vi "Save Enabled Settings.vi"(8 "Error in":errorcluster caption="Error in (no error)", 10 "Enabled Sections":T1={"Projects"=TRUE, "Interfaces"=TRUE, "Classes"=TRUE, "Libraries"=TRUE, "VIs"=TRUE, "Controls"=TRUE, "LLBs"=TRUE}, 11 "Settings Path":path) -> (0 "Error out":errorcluster)   [LabVIEW 2023, in "VIDoc Printer.lvlib" / "Printer Settings.lvclass"]
uses:
  Printer Settings.lvclass
  Enabled Sections Cluster.ctl
  55d7a2f0-e96c-4448-af12-77755b1bcd60.vi
  <vilib>/JDP Science/JSONtext/Variant to JSON Text.vi
  <vilib>/JDP Science/JSONtext/LVClass Serializer/JSONtext LVClass Serializer.lvclass
  VIDoc Settings/VIDoc Settings.lvclass
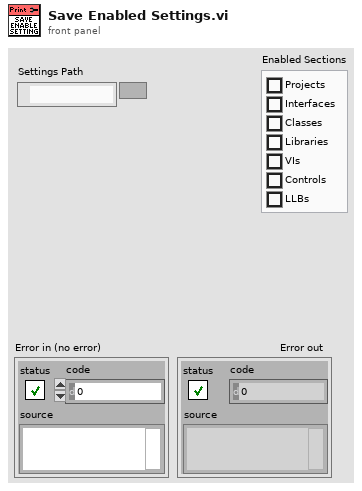
[diagram p1: front panel]
types:
  T1 = typedef "VIDoc Printer.lvlib/Printer Settings.lvclass/Enabled Sections Cluster.ctl" = cluster{"Projects":bool, "Interfaces":bool, "Classes":bool, "Libraries":bool, "VIs":bool, "Controls":bool, "LLBs":bool}
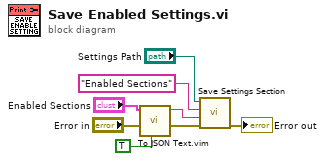
[diagram p0: block diagram]
diagram:
  n1 = call "To JSON Text.vim"("Pretty Print?"=TRUE, "error in (no error)"="Error in", "Anything"="Enabled Sections") -> ("error out"=w7:errorcluster, "<JSON>"=w5:string)  [unwired: 7 in]
  n2 = call "Save Settings Section.vi"("Error in"=w7, "JSON Object"=w5, "Section Name"="Enabled Sections", "JSON Settings Path"="Settings Path") -> ("Error out"=→"Error out":errorcluster)  [unwired: 7 in]
